vi "USB6343_Control_v1.2.vi"(9 "event rsg handle":refnum<event-registration>) -> ()   [LabVIEW 2013]
uses:
  <vilib>/DAQmx/write.llb/DAQmx Write.vi
  <vilib>/DAQmx/write.llb/DAQmx Write (Digital 1D Bool NChan 1Samp 1Line).vi
  <vilib>/DAQmx/write.llb/DAQmx Write (Analog 1D DBL NChan 1Samp).vi
  <vilib>/DAQmx/read.llb/DAQmx Read.vi
  <vilib>/DAQmx/read.llb/DAQmx Read (Analog 1D DBL NChan 1Samp).vi
  <vilib>/DAQmx/miscellaneous.llb/DAQmx Fill In Error Info.vi
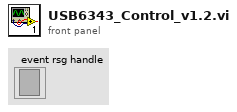
[diagram p1: front panel]
types:
  T1 = cluster{"AI Task":refnum<k21>, "AO Task":refnum<k21>, "DO Task":refnum<k21>, "DI Task":refnum<k21>}
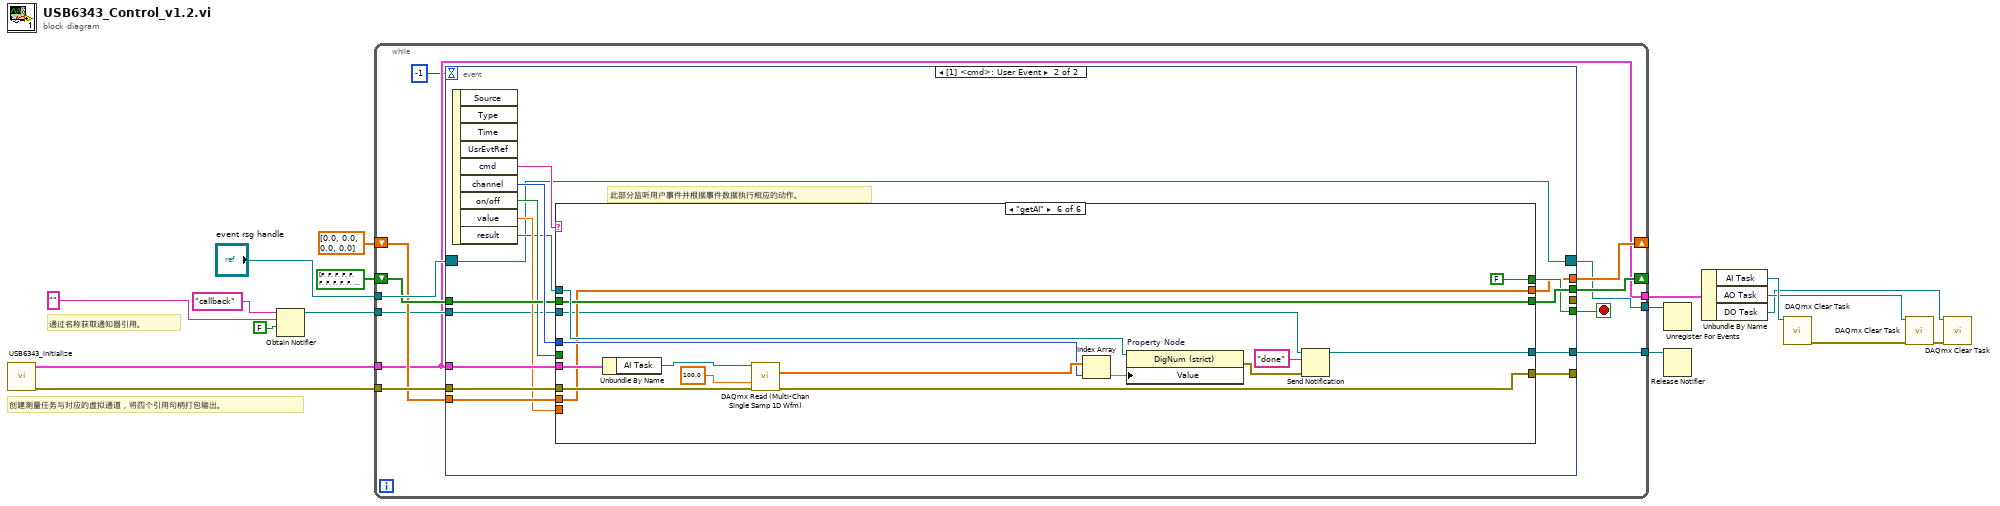
[diagram p0: block diagram]
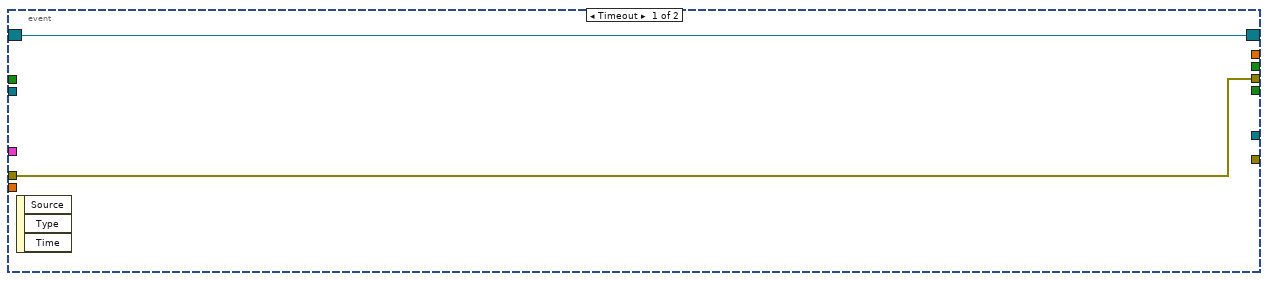
[diagram p2: hidden frame]
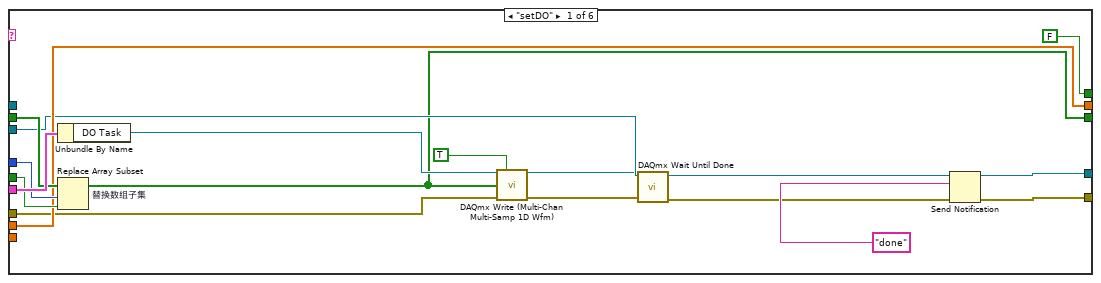
[diagram p3: hidden frame]
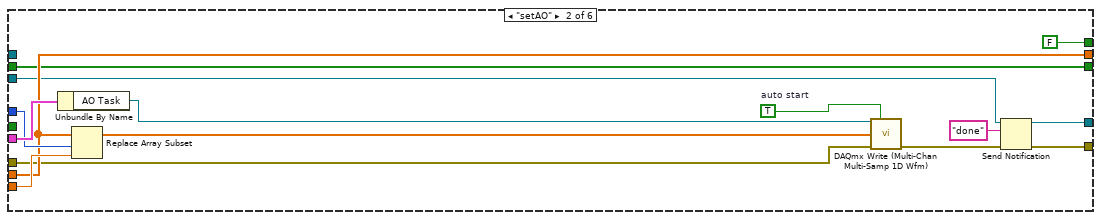
[diagram p4: hidden frame]
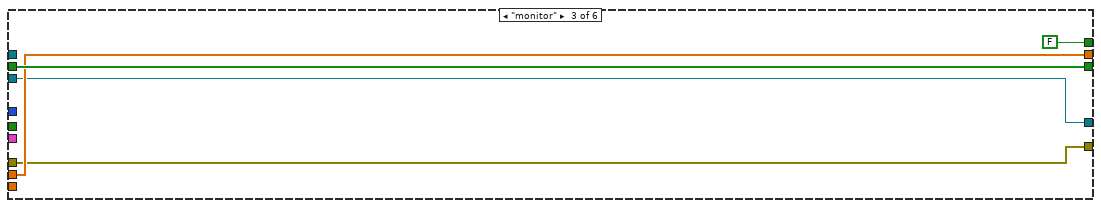
[diagram p5: hidden frame]
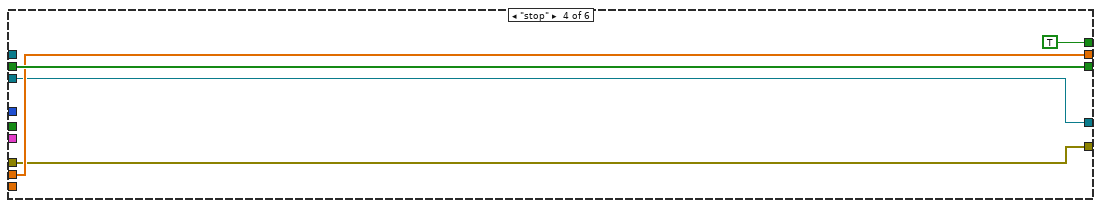
[diagram p6: hidden frame]
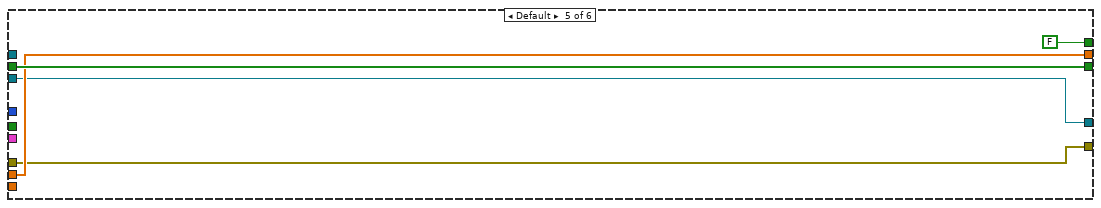
[diagram p7: hidden frame]
diagram:
  # "通过名称获取通知器引用。"
  # "创建测量任务与对应的虚拟通道，将四个引用句柄打包输出。"
  n1 = call "USB6343_initialize.vi"() -> ("error out"=w17:errorcluster, "tasks"=w6:T1)  [unwired: 10 in]
  n2 = Obtain Notifier(name (unnamed)="callback" ("名称（未命名）"), notification data type="", create if not found? (T)=FALSE ("如未找到是否创建？(T)")) -> (notifier out=w8:refnum<notifier>)  [unwired: 1 in, 2 out]
  n3 = while {
    tunnel: w6 -> [w19]
    tunnel: w17 -> [w29]
    tunnel: "event rsg handle" -> [w28]
    shift-right: [w26] -> _
    shift-left: bool[] [FALSE, FALSE, FALSE, FALSE, FALSE, FALSE, FALSE, FALSE, FALSE, FALSE, FALSE, FALSE, FALSE, FALSE, FALSE, FALSE] -> [w27]
    shift-right: [w23] -> _
    shift-left: dbl[] [0.0, 0.0, 0.0, 0.0] ("data") -> [w24]
    tunnel: [w22] -> w12
    tunnel: w8 -> [w21]
    tunnel: [w20] -> w7
    tunnel: [w19] -> w4
    stop <- w25 stop-if-true
    n4 = event shown="[1] <cmd>: User Event" {
      selector: w28 -> [w30 w34]
      dyn-events: [w30 w34] -> w22
      timeout: -1 -> [_ _]
      tunnel: w19 -> [_ w46]
      tunnel: [w31 _] -> _
      tunnel: w29 -> [w31 w45]
      tunnel: w27 -> [_ w44]
      tunnel: [_ w42] -> w26
      tunnel: [_ w40] -> w25
      tunnel: w24 -> [_ w39]
      tunnel: [_ w37] -> w23
      tunnel: [_ w35] -> _
      tunnel: w21 -> [_ w33]
      tunnel: [_ w32] -> w20
      event Timeout {
        n5 = event-data() -> ()  [unwired: 1 in, 3 out]
      }
      event User Event {
        # "此部分监听用户事件并根据事件数据执行相应的动作。"
        n6 = event-data() -> ("cmd"=w41:string, "channel"=w47:i32, "on/off"=w43:bool, "value"=w38:dbl, "result"=w36:refnum<vi>)  [unwired: 1 in, 4 out]
        n7 = case shown="\"getAI\"" w41 {
          tunnel: w47 -> [w62 w77 _ _ _ w104]
          tunnel: w46 -> [w64 w79 _ _ _ w110]
          tunnel: w45 -> [w54 w70 w81 w86 w91 w106]
          tunnel: w44 -> [w63 w74 w84 w89 w94 w102]
          tunnel: w43 -> [w61 _ _ _ _ _]
          tunnel: [w52 w74 w84 w89 w94 w102] -> w42
          tunnel: [FALSE FALSE FALSE TRUE FALSE FALSE] -> w40
          tunnel: w39 -> [w59 w75 w83 w87 w92 w101]
          tunnel: w38 -> [_ w76 _ _ _ _]
          tunnel: [w59 w75 w83 w87 w92 w101] -> w37
          tunnel: w36 -> [_ _ _ _ _ w108]
          tunnel: [w58 w68 w81 w86 w91 w99] -> w35
          tunnel: w33 -> [w57 w66 w80 w85 w90 w98]
          tunnel: [w55 w67 w80 w85 w90 w97] -> w32
          frame "setDO" {
            n8 = Unbundle By Name(w64) -> ("DO Task"=w53:refnum<k21>)
            n9 = Replace Array Subset "替换数组子集"(array=w63, new element=w61, index=w62) -> (w52:bool[])
            n10 = call-poly "DAQmx Write (Multi-Chan Multi-Samp 1D Wfm).vi"("task/channels in"=w53, "auto start"=TRUE, "data"=w52, "error in"=w54) -> ("task out"=w48:refnum<k21>, "error out"=w50:errorcluster)  [unwired: 9 in, 1 out]
            n11 = call <vilib>:"DAQmx Wait Until Done.vi"("task/channels in"=w48, "error in"=w50) -> ("error out"=w49:errorcluster)  [unwired: 12 in, 1 out]
            n12 = Send Notification(notification="done" ("通知"), notifier=w57, error in (no error)=w49) -> (notifier out=w55:refnum<notifier>, error out=w58:errorcluster)
          }
          frame "setAO" {
            w72 = TRUE  # auto start
            n13 = Unbundle By Name(w79) -> ("AO Task"=w78:refnum<k21>)
            n14 = Replace Array Subset(array=w75, new element=w76, index=w77) -> (w73:dbl[])
            n15 = call-poly "DAQmx Write (Multi-Chan Multi-Samp 1D Wfm).vi"("task/channels in"=w78, "auto start"=w72, "data"=w73, "error in"=w70) -> ("error out"=w69:errorcluster)  [unwired: 9 in, 2 out]
            n16 = Send Notification(notification="done" ("通知"), notifier=w66, error in (no error)=w69) -> (notifier out=w67:refnum<notifier>, error out=w68:errorcluster)
          }
          frame "monitor" {
          }
          frame "stop" {
          }
          frame Default {
          }
          frame "getAI" {
            n17 = Unbundle By Name(w110) -> ("AI Task"=w109:refnum<k21>)
            n18 = call-poly "DAQmx Read (Multi-Chan Single Samp 1D Wfm).vi"("task/channels in"=w109, "timeout"=100.0, "error in"=w106) -> ("data"=w105:dbl[], "error out"=w99:errorcluster)  [unwired: 10 in, 1 out]
            n19 = Index Array(array=w105, index=w104) -> (element=w103:dbl)
            n20 = property on="Property Node" class="DigNum (strict)"(reference=w108, "Value"=w103) -> (error out=w95:errorcluster)  [unwired: 1 in, 1 out]
            n21 = Send Notification(notification="done" ("通知"), notifier=w98, error in (no error)=w95) -> (notifier out=w97:refnum<notifier>)  [unwired: 1 out]
          }
        }
      }
    }
  }
  n22 = Unregister For Events(event registration refnum=w12) -> ()  [unwired: 1 in, 1 out]
  n23 = Release Notifier(notifier=w7) -> ()  [unwired: 2 in, 3 out]
  n24 = Unbundle By Name(w4) -> ("AI Task"=w16:refnum<k21>, "AO Task"=w15:refnum<k21>, "DO Task"=w14:refnum<k21>)
  n25 = call <vilib>:"DAQmx Clear Task.vi"("task in"=w16) -> ("error out"=w3:errorcluster)  [unwired: 14 in]
  n26 = call <vilib>:"DAQmx Clear Task.vi"("task in"=w15, "error in"=w3) -> ("error out"=w2:errorcluster)  [unwired: 13 in]
  n27 = call <vilib>:"DAQmx Clear Task.vi"("task in"=w14, "error in"=w2) -> ()  [unwired: 13 in, 1 out]
